vi "BLDCMotorOpen.vi"(4 "Timeout (mSec)":i32=5000, 6 "Connection":u16(ring) items=["No Preference", "Remote", "Local"], 8 "error in":errorcluster, 11 "Device Info":T1={"Serial Number"=-1, "Channel"=0, "Port"=0}) -> (0 "error out":errorcluster, 1 "Attached?":bool, 2 "Serial Number Return":i32, 3 "Phidget ID":u64)   [LabVIEW 2012, in "Phidget BLDC Motor.lvlib"]
doc: "${BLDCMotor:OpenHeader}"
uses:
  <instrlib>/Phidgets/Phidget BLDC Motor/Phidget BLDC Motor.lvlib
  <instrlib>/Phidgets/Phidget Common/Phidget Common.lvlib
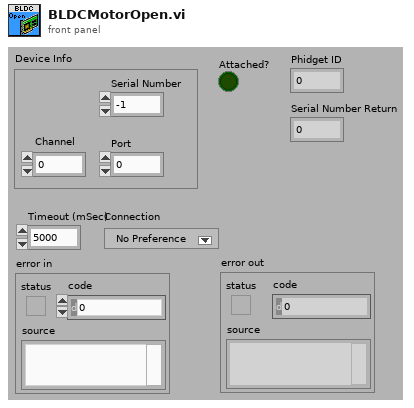
[diagram p1: front panel]
types:
  T1 = cluster{"Serial Number":i32, "Channel":i32, "Port":i32}
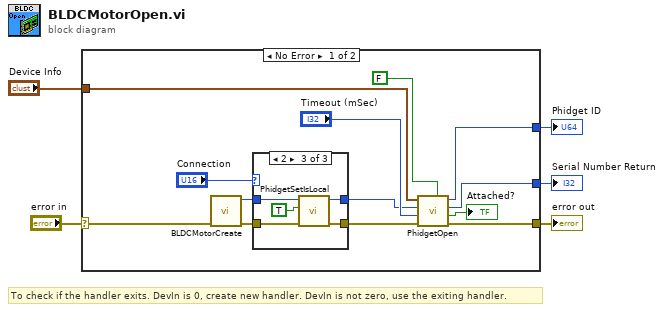
[diagram p0: block diagram]
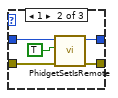
[diagram p3: hidden frame]
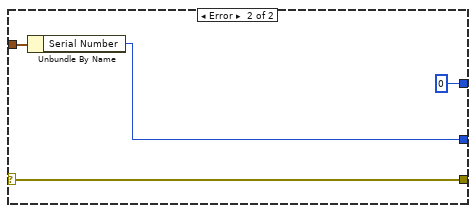
[diagram p4: hidden frame]
diagram:
  # "To check if the handler exits. DevIn is 0, create new handler. DevIn is not zero, use the exiting handler."
  n1 = case shown="No Error" "error in" {
    selector: "error in" -> [w8 w34]
    tunnel: [w17 w34] -> w4
    tunnel: "Device Info" -> [w14 w32]
    tunnel: [w15 0 ("Device Out")] -> w2
    tunnel: [w13 w31] -> w1
    frame No Error {
      n2 = call <instrlib>:"BLDCMotorCreate.vi"("error in"=w8) -> ("error out"=w7:errorcluster, "Device Out"=w6:u64)  [unwired: 9 in]
      n3 = case shown="2" "Connection" {
        tunnel: w6 -> [w20 w25 w27]
        tunnel: w7 -> [w19 w24 w30]
        tunnel: [w19 w21 w29] -> w11
        tunnel: [w20 w22 w28] -> w10
        frame 0, Default {
        }
        frame 1 {
          n4 = call <instrlib>:"PhidgetSetIsRemote.vi"("error in"=w24, "Remote"=TRUE, "Device In"=w25) -> ("error out"=w21:errorcluster, "Device Out"=w22:u64)  [unwired: 7 in]
        }
        frame 2 {
          n5 = call <instrlib>:"PhidgetSetIsLocal.vi"("error in"=w30, "Local"=TRUE, "Device In"=w27) -> ("error out"=w29:errorcluster, "Device Out"=w28:u64)  [unwired: 7 in]
        }
      }
      n6 = call <instrlib>:"PhidgetOpen.vi"("IsHubPort"=FALSE, "error in"=w11, "millis"="Timeout (mSec)", "Phidget ID"=w10, "Device Info"=w14) -> ("error out"=w17:errorcluster, "Attached?"=→"Attached?":bool, "Serial Number Return"=w13:i32, "Device Out"=w15:u64)  [unwired: 3 in]
    }
    frame Error {
      n7 = Unbundle By Name(w32) -> ("Serial Number"=w31:i32)
    }
  }
  "error out" <- w4
  "Phidget ID" <- w2
  "Serial Number Return" <- w1
